vi "Get_Variant_Strings_from_Enum.vi"(8 "error in (no error)":errorcluster, 11 "Enum":variant) -> (0 "error out":errorcluster, 1 "String value":string, 2 "Enum name":string, 3 "Enum strings":string[](array[string]))   [LabVIEW 2012]
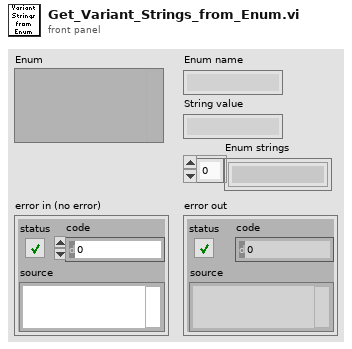
[diagram p1: front panel]
types:
  T1 = cluster{"length":u16, "private":u8, "type":enum8{"<Null>", "I8", "I16", "I32", "I64", "U8", "U16", "U32", "U64", "SGL", "DBL", "EXT", "CSG", "CDB", "CXT", "0x0F", "0x10", "0x11", "0x12", "0x13", "0x14", "Enum U8", "Enum U16", "Enum U32", "Enum U64", "SGL PQ", "DBL PQ", "EXT PQ", "CSG PQ", "CDB PQ", "CXT PQ", "0x1F", "0x20", "Boolean", "0x22", "0x23", "0x24", "0x25", "0x26", "0x27", "0x28", "0x29", "0x2A", "0x2B", "0x2C", "0x2D", "0x2E", "0x2F", "String", "0x31", "Path", "Pict", "0x34", "0x35", "0x36", "DAQ", "0x38", "0x39", "0x3A", "0x3B", "0x3C", "0x3D", "0x3E", "0x3F", "Array", "0x41", "0x42", "0x43", "0x44", "0x45", "0x46", "0x47", "0x48", "0x49", "0x4A", "0x4B", "0x4C", "0x4D", "0x4E", "0x4F", "Cluster", "0x51", "0x52", "Variant", "Waveform", "0x55", "0x56", "0x57", "0x58", "0x59", "0x5A", "0x5B", "0x5C", "0x5D", "0x5E", "0x5F", "0x60", "0x61", "0x62", "0x63", "0x64", "0x65", "0x66", "0x67", "0x68", "0x69", "0x6A", "0x6B", "0x6C", "0x6D", "0x6E", "0x6F", "Refnum"}, "# elements":u16}
  T2 = enum8{"<Null>", "I8", "I16", "I32", "I64", "U8", "U16", "U32", "U64", "SGL", "DBL", "EXT", "CSG", "CDB", "CXT", "0x0F", "0x10", "0x11", "0x12", "0x13", "0x14", "Enum U8", "Enum U16", "Enum U32", "Enum U64", "SGL PQ", "DBL PQ", "EXT PQ", "CSG PQ", "CDB PQ", "CXT PQ", "0x1F", "0x20", "Boolean", "0x22", "0x23", "0x24", "0x25", "0x26", "0x27", "0x28", "0x29", "0x2A", "0x2B", "0x2C", "0x2D", "0x2E", "0x2F", "String", "0x31", "Path", "Pict", "0x34", "0x35", "0x36", "DAQ", "0x38", "0x39", "0x3A", "0x3B", "0x3C", "0x3D", "0x3E", "0x3F", "Array", "0x41", "0x42", "0x43", "0x44", "0x45", "0x46", "0x47", "0x48", "0x49", "0x4A", "0x4B", "0x4C", "0x4D", "0x4E", "0x4F", "Cluster", "0x51", "0x52", "Variant", "Waveform", "0x55", "0x56", "0x57", "0x58", "0x59", "0x5A", "0x5B", "0x5C", "0x5D", "0x5E", "0x5F", "0x60", "0x61", "0x62", "0x63", "0x64", "0x65", "0x66", "0x67", "0x68", "0x69", "0x6A", "0x6B", "0x6C", "0x6D", "0x6E", "0x6F", "Refnum"}
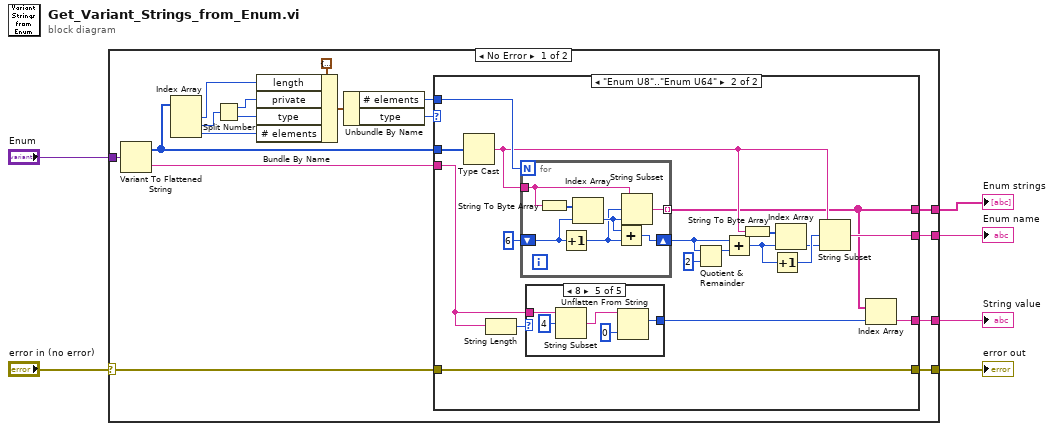
[diagram p0: block diagram]
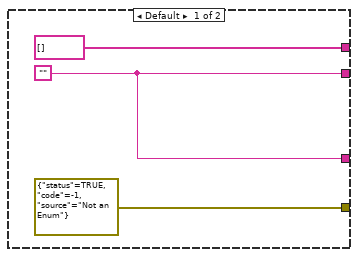
[diagram p2: hidden frame]
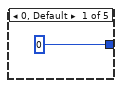
[diagram p3: hidden frame]
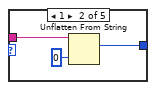
[diagram p4: hidden frame]
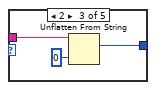
[diagram p5: hidden frame]
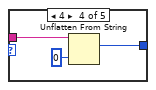
[diagram p6: hidden frame]
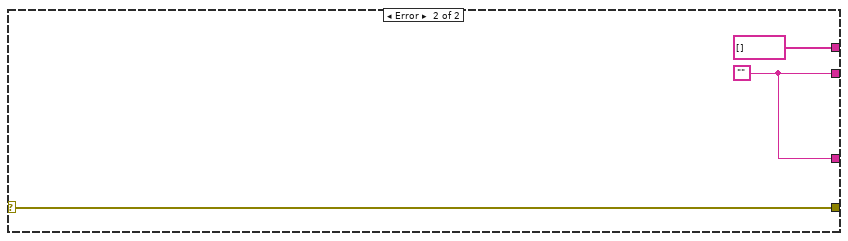
[diagram p7: hidden frame]
diagram:
  n1 = case shown="No Error" "error in (no error)" {
    selector: "error in (no error)" -> [w18 w69]
    tunnel: [w23 w69] -> w5
    tunnel: [w21 string[] [] ("enum strings")] -> w2
    tunnel: [w20 w68] -> w4
    tunnel: [w19 w68] -> w3
    tunnel: "Enum" -> [w17 _]
    frame No Error {
      n2 = Variant To Flattened String(Variant=w17) -> (data string=w16:string, 1:w9:i16[])
      n3 = Index Array(array=w9) -> (element #1=w11:i16, element #2=w14:i16, element #3=w15:i16)  [unwired: 3 in]
      n4 = Split Number(x=w14) -> (hi(x)=w12:u8, lo(x)=w13:u8)
      n5 = Bundle By Name(cluster=T1 {"length"=0, "private"=0, "type"=enum."<Null>", "# elements"=0} ("Type Descriptor Header"), "length"=w11, "private"=w12, "type"=w13, "# elements"=w15) -> (w8:T1)
      n6 = Unbundle By Name(w8) -> ("# elements"=w7:u16, "type"=w22:T2)
      n7 = case shown="\"Enum U8\"..\"Enum U64\"" w22 {
        tunnel: [errorcluster {"status"=TRUE, "code"=-1, "source"="Not an Enum"} ("error out") w27] -> w23
        tunnel: w9 -> [_ w40]
        tunnel: w16 -> [_ w43]
        tunnel: [string[] [] w28] -> w21
        tunnel: [w24 w29] -> w20
        tunnel: [w24 w41] -> w19
        tunnel: w18 -> [_ w27]
        tunnel: w7 -> [_ w39]
        frame Default {
          w24 = ""
        }
        frame "Enum U8".."Enum U64" {
          n8 = Type Cast(x=w40) -> (*(type *) &x=w30:string)  [unwired: 1 in]
          n9 = String Length(string=w43) -> (length=w44:i32)
          n10 = for {
            N: w39 -> [_]
            shift-right: [w45] -> w38
            shift-left: 6 -> [w47]
            tunnel: [w46] -> w28 mode=indexing
            tunnel: w30 -> [w48]
            n11 = String To Byte Array(string=w48) -> (unsigned byte array=w49:u8[])
            n12 = Increment(x=w47) -> (x+1=w50:i32)
            n13 = Index Array(array=w49, index=w47) -> (element=w51:u8)
            n14 = Add(x=w51, y=w50) -> (x+y=w45:i32)
            n15 = String Subset(string=w48, offset (0)=w50, length (rest)=w51) -> (substring=w46:string)
          }
          n16 = case shown="8" w44 {
            tunnel: w43 -> [_ w55 w58 w61 w62]
            tunnel: [u32 0 ("U32") w53 w56 w59 w65] -> w42
            frame 0, Default {
            }
            frame 1 {
              n17 = Unflatten From String(type=u8 0, binary string=w55) -> (value=w53:u8)  [unwired: 3 in, 2 out]
            }
            frame 2 {
              n18 = Unflatten From String(type=u16 0, binary string=w58) -> (value=w56:u16)  [unwired: 3 in, 2 out]
            }
            frame 4 {
              n19 = Unflatten From String(type=u32 0, binary string=w61) -> (value=w59:u32)  [unwired: 3 in, 2 out]
            }
            frame 8 {
              n20 = String Subset(string=w62, offset (0)=4) -> (substring=w63:string)  [unwired: 1 in]
              n21 = Unflatten From String(type=u32 0, binary string=w63) -> (value=w65:u32)  [unwired: 3 in, 2 out]
            }
          }
          n22 = Quotient & Remainder(x=w38, y=2) -> (x-y*floor(x/y)=w37:i32)  [unwired: 1 out]
          n23 = Add(x=w38, y=w37) -> (x+y=w31:i32)
          n24 = String To Byte Array(string=w30) -> (unsigned byte array=w34:u8[])
          n25 = Increment(x=w31) -> (x+1=w33:i32)
          n26 = Index Array(array=w34, index=w31) -> (element=w32:u8)
          n27 = String Subset(string=w30, offset (0)=w33, length (rest)=w32) -> (substring=w29:string)
          n28 = Index Array(array=w28, index=w42) -> (element=w41:string)
        }
      }
    }
    frame Error {
      w68 = ""
    }
  }
  "error out" <- w5
  "Enum name" <- w4
  "String value" <- w3
  "Enum strings" <- w2
